vi "6_array.vi"() -> ()   [LabVIEW 2017]
panel:
  out "iterações":dbl[](array[numeric])
  in  "multiplicador":dbl
  in  "length":i32
  in  "index":i32
  out "arranjo final":dbl[](array[numeric])
  out "arranjo resultante":dbl[](array[numeric])
  out "arranjo inicial":dbl[](array[numeric])
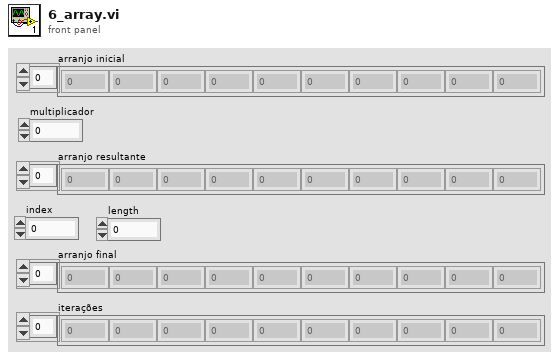
[diagram p1: front panel]
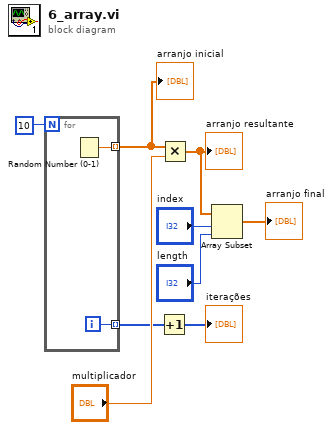
[diagram p0: block diagram]
diagram:
  n1 = for {
    N: 10 -> [_]
    tunnel: [w11] -> w1 mode=indexing
    tunnel: [w10] -> w3 mode=indexing
    i -> [w10]
    n2 = Random Number (0-1)() -> (number: 0 to 1=w11:dbl)
  }
  "arranjo inicial" <- w1
  n3 = Increment(x=w3) -> (x+1=→"iterações":i32[])
  n4 = Multiply(x=w1, y="multiplicador") -> (x*y=w8:dbl[])
  "arranjo resultante" <- w8
  n5 = Array Subset(array=w8, index="index", length="length") -> (→"arranjo final":dbl[])
